vi "zipEpub.vi"(4 "线程":i32, 6 "删除临时文件":bool, 8 "error in (no error)":errorcluster caption="错误输入（无错误）", 11 "EPUB 输入":refnum<class "EPUB.lvclass">) -> (0 "error out":errorcluster caption="错误输出", 3 "EPUB 输出":refnum<class "EPUB.lvclass">)   [LabVIEW 2016, in "EPUB.lvclass"]
uses:
  EPUB.lvclass
  EPUB.lvclass/EPUB.ctl
  <userlib>/_OpenG.lib/lvzip/lvzip.llb/ZLIB Open Zip Archive__ogtk.vi
  <userlib>/_OpenG.lib/lvzip/lvzip.llb/ZLIB Store File__ogtk.vi
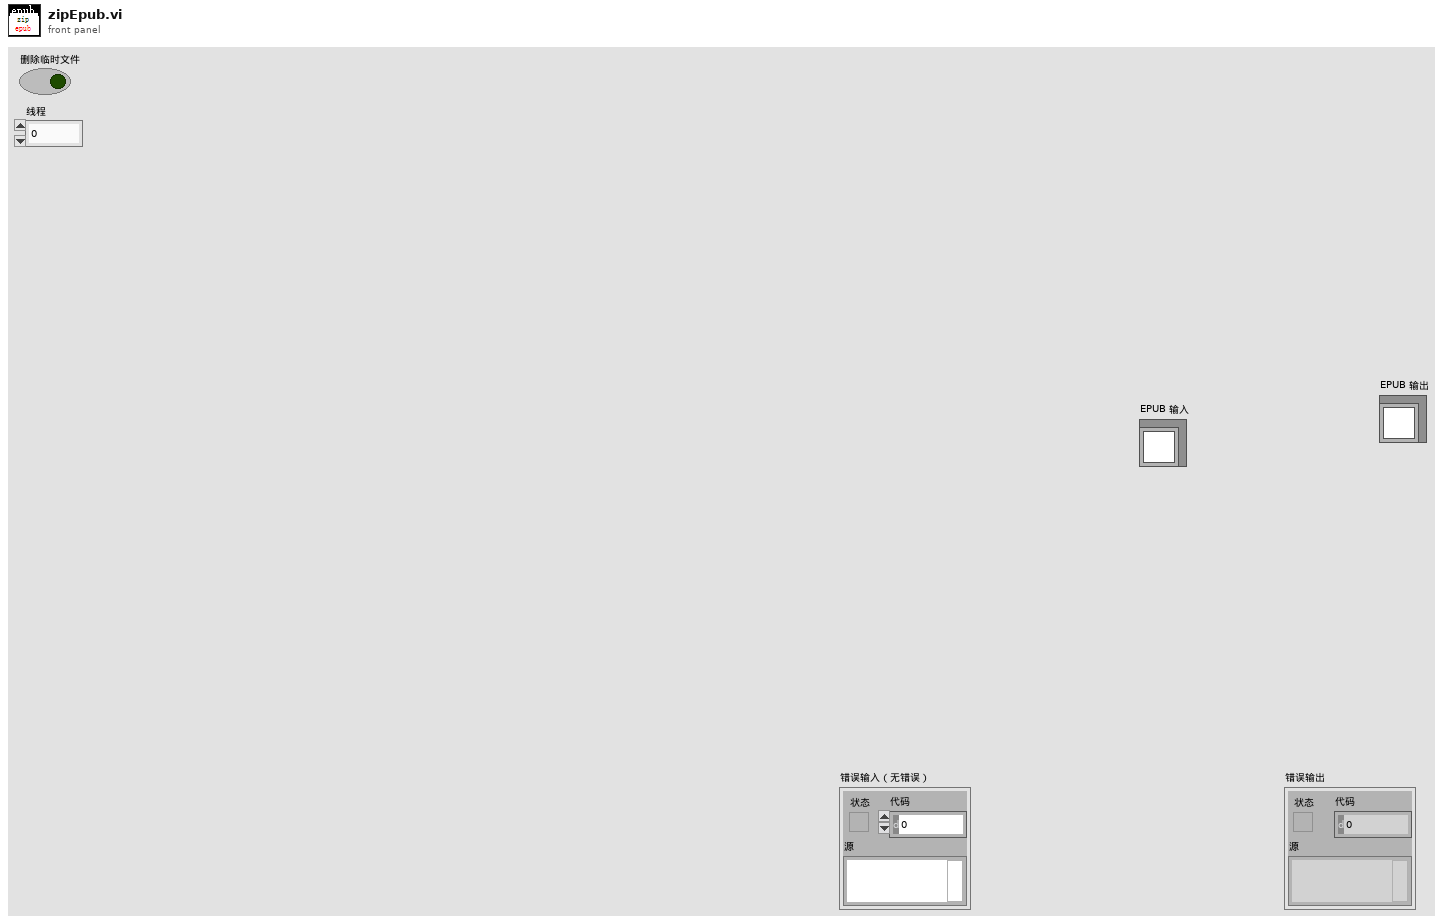
[diagram p1: front panel]
types:
  T1 = typedef "ZLIB Zip Handle__ogtk.ctl" = refnum<k1>
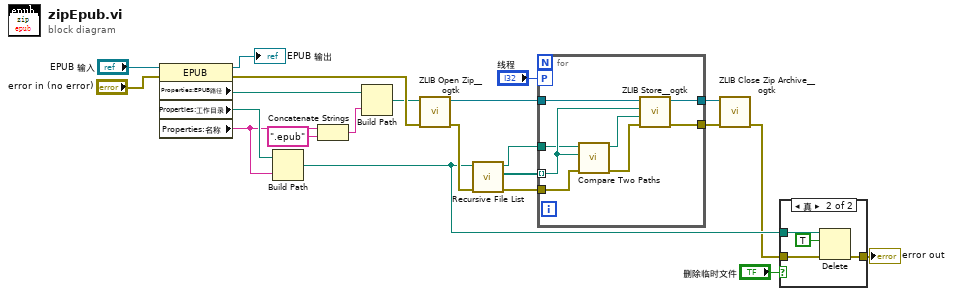
[diagram p0: block diagram]
diagram:
  n1 = property class="EPUB"(reference="EPUB 输入", error in="error in (no error)") -> (reference out=→"EPUB 输出":refnum<class "EPUB.lvclass">, error out=w4:errorcluster, "Properties:EPUB路径"=w21:path, "Properties:工作目录"=w18:path, "Properties:名称"=w17:string)
  n2 = Build Path(base path=w18, name or relative path=w17) -> (appended path=w8:path)
  n3 = Concatenate Strings(w17, ".epub" ("字符串")) -> (w20:string)
  n4 = Build Path(base path=w21, name or relative path=w20) -> (appended path=w3:path)
  n5 = call-poly <userlib>:"ZLIB Open Zip__ogtk.vi"("error in (no error)"=w4, "archive name"=w3) -> ("error out"=w16:errorcluster, "zip Refnum"=w2:T1)  [unwired: 3 in, 1 out]
  n6 = call <vilib>:"Recursive File List.vi"("error in (no error)"=w16, "Folder Path"=w8) -> ("error out"=w13:errorcluster, "All Files in Dir"=w15:path[], "dup Folder Path"=w14:path)  [unwired: 5 in, 2 out]
  n7 = for {
    tunnel: w15 -> [w28] mode=indexing
    tunnel: w13 -> [w25]
    tunnel: [w29] -> w12
    tunnel: w14 -> [w27]
    workers-P: "线程" -> [_]
    tunnel: [w30] -> w1
    tunnel: w2 -> [w23]
    n8 = call <vilib>:"Compare Two Paths.vi"("error in (no error)"=w25, "Path 2"=w28, "Path 1"=w27) -> ("error out"=w24:errorcluster, "Relative Path from 1 to 2"=w26:path)  [unwired: 5 in, 2 out]
    n9 = call-poly <userlib>:"ZLIB Store__ogtk.vi"("error in (no error)"=w24, "internal name (same as source name)"=w26, "source path"=w28, "zip Refnum"=w23) -> ("error out"=w29:errorcluster, "zip Refnum out"=w30:T1)  [unwired: 6 in]
  }
  n10 = call <userlib>:"ZLIB Close Zip Archive__ogtk.vi"("error in (no error)"=w12, "zip Refnum"=w1) -> ("error out"=w6:errorcluster)  [unwired: 4 in, 1 out]
  n11 = case shown="真" "删除临时文件" {
    tunnel: w6 -> [w31 w35]
    tunnel: [w31 w34] -> w9
    tunnel: w8 -> [_ w33]
    frame False {
    }
    frame True {
      n12 = Delete(path (use dialog)=w33, entire hierarchy (F)=TRUE ("整个层次结构(F)"), error in=w35) -> (error out=w34:errorcluster)  [unwired: 2 in, 2 out]
    }
  }
  "error out" <- w9
